vi "Get Camera Class.vi"(11 "Device Type":T1) -> (3 "Specific Class Reference":refnum<class "Camera.lvclass">)   [LabVIEW 2011, in "Image UDP Broadcast Custom Device.lvlib"]
uses:
  Image UDP Broadcast Custom Device.lvlib
  Configuration/Ctls/Device Type.ctl
  Camera Class/Camera.lvclass
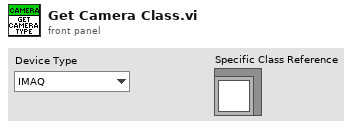
[diagram p1: front panel]
types:
  T1 = typedef "Image UDP Broadcast Custom Device.lvlib/Device Type.ctl" = enum8{"IMAQ", "IMAQdx"}
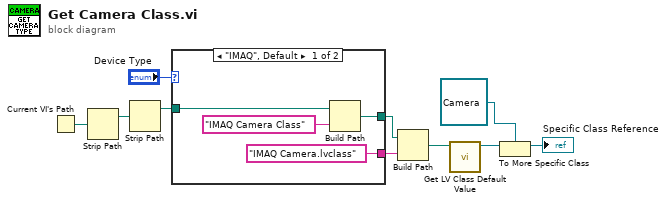
[diagram p0: block diagram]
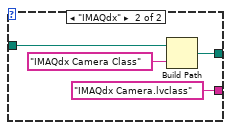
[diagram p2: hidden frame]
diagram:
  n1 = Current VI's Path() -> (path=w10:path)
  n2 = Strip Path(path=w10) -> (stripped path=w4:path)  [unwired: 1 out]
  n3 = Strip Path(path=w4) -> (stripped path=w3:path)  [unwired: 1 out]
  n4 = case shown="\"IMAQ\", Default" "Device Type" {
    tunnel: ["IMAQ Camera.lvclass" ("name or relative path") "IMAQdx Camera.lvclass" ("name or relative path")] -> w5
    tunnel: w3 -> [w14 w18]
    tunnel: [w12 w15] -> w2
    frame "IMAQ", Default {
      n5 = Build Path(base path=w14, name or relative path="IMAQ Camera Class") -> (appended path=w12:path)
    }
    frame "IMAQdx" {
      n6 = Build Path(base path=w18, name or relative path="IMAQdx Camera Class") -> (appended path=w15:path)
    }
  }
  n7 = Build Path(base path=w2, name or relative path=w5) -> (appended path=w1:path)
  n8 = call <vilib>:"Get LV Class Default Value.vi"("class path"=w1) -> ("object"=w9:refnum<class>)  [unwired: 9 in, 1 out]
  n9 = To More Specific Class(target class=refnum<class "Camera.lvclass"> refnum ("Image UDP Broadcast Custom Device.lvlib:Camera.lvclass"), reference=w9) -> (specific class reference=→"Specific Class Reference":refnum<class "Camera.lvclass">)  [unwired: 1 in, 1 out]
